vi "test_libssh2_crypto_engine.vi"() -> ()   [LabVIEW 2013, in "libssh2_tests.lvlib"]
uses:
  libssh2_tests.lvlib
  libssh2/libssh2_crypto_engine.ctl
  libssh2/libssh2_init_default.vi
  libssh2/libssh2.lvlib
  <vilib>/addons/_JKI Toolkits/Caraya/classes/Test/Test.lvclass
  <vilib>/addons/_JKI Toolkits/Caraya/classes/Assert/Assert.lvclass
panel:
  out "error out":errorcluster
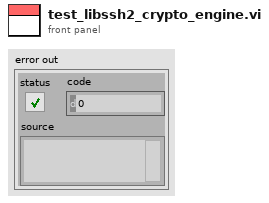
[diagram p1: front panel]
types:
  T1 = typedef "libssh2.lvlib/libssh2_crypto_engine.ctl" = enum16{"no crypto", "OpenSSL", "gcrypt", "mbedTLS", "WinCNG", "OS400qc3"}
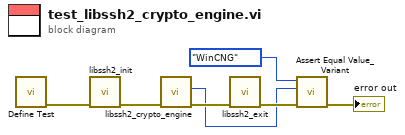
[diagram p0: block diagram]
diagram:
  n1 = call <vilib>:"Define Test.vi"() -> ("error out"=w3:errorcluster)  [unwired: 10 in, 1 out]
  n2 = call-poly "libssh2_init.vi"("error in (no error)"=w3) -> ("error out"=w7:errorcluster)  [unwired: 10 in]
  n3 = call "libssh2_crypto_engine.vi"("error in (no error)"=w7) -> ("error out"=w5:errorcluster, "crypto engine"=w2:T1)  [unwired: 9 in]
  n4 = call "libssh2_exit.vi"("error in (no error)"=w5) -> ("error out"=w6:errorcluster)  [unwired: 10 in]
  n5 = call <vilib>:"Assert Equal Value_Variant.vi"("error in (no error)"=w6, "Y"=w2, "X"=libssh2_crypto_engine."WinCNG" ("crypto engine")) -> ("error out"=→"error out":errorcluster)  [unwired: 7 in, 1 out]
